vi "Pot Modules.vi"(7 "Console Log in":refnum<class "Console Log.lvclass">, 8 "error in":errorcluster, 11 "Potting Procedure in":refnum<class "Potting Procedure.lvclass">) -> (0 "error out":errorcluster, 3 "Potting Procedure out":refnum<class "Potting Procedure.lvclass">, 5 "Console Log out":refnum<class "Console Log.lvclass">)   [LabVIEW 2011, in "Potting Procedure.lvclass"]
uses:
  Potting Procedure.lvclass
  Application Utilities/Console Log/Console Log.lvclass
  Shared Components/SyringeTool Class/SyringeTool Class.lvclass
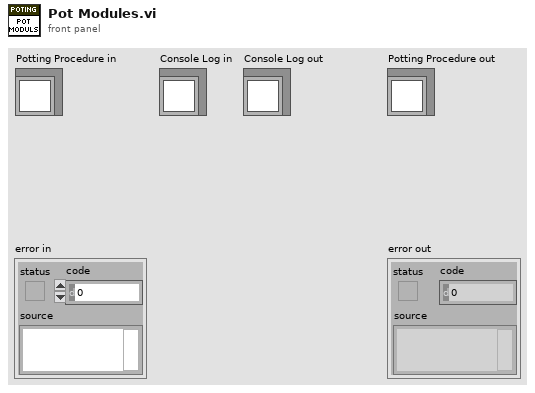
[diagram p1: front panel]
types:
  T1 = typedef "Module Potting Data.ctl" = cluster{"HDI Bond Pad Groups":T2[], "BBM Bond Pad Groups":T2[], "TBM - TBM Side":T2[], "TBM - HDI Side":T2[], "Address Pads":T2[], "Chuck":i32, "Slot":i32, "HV - HDI":T3, "HV - BBM":T3}
  T2 = typedef "3d Line.ctl" = cluster{"Start":refnum<class "Vec3d Class.lvclass">, "End":refnum<class "Vec3d Class.lvclass">, "Enable":bool}
  T3 = typedef "3d Point.ctl" = cluster{"Point":refnum<class "Vec3d Class.lvclass">, "Enable":bool}
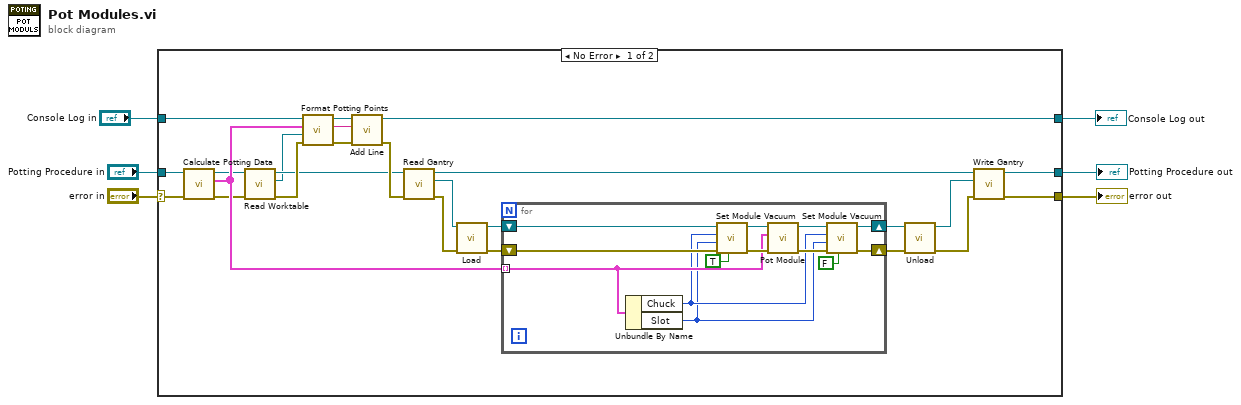
[diagram p0: block diagram]
diagram:
  n1 = case shown="No Error" "error in" {
    selector: "error in" -> [w20 w47]
    tunnel: [w19 w47] -> w5
    tunnel: [w21 w46] -> w3
    tunnel: "Potting Procedure in" -> [w31 w46]
    tunnel: "Console Log in" -> [w18 w45]
    tunnel: [w13 w45] -> w1
    frame No Error {
      n2 = call "Calculate Potting Data.vi"("error in"=w20, "Potting Procedure in"=w31) -> ("error out"=w10:errorcluster, "Module Potting Data"=w17:T1[], "Potting Procedure out"=w11:refnum<class "Potting Procedure.lvclass">)  [unwired: 7 in]
      n3 = call-dynamic "Read Worktable.vi"("error in"=w10, "Potting Procedure in"=w11) -> ("error out"=w9:errorcluster, "WorkTable out"=w7:refnum<class "WorkTable Class.lvclass">, "Potting Procedure out"=w8:refnum<class "Potting Procedure.lvclass">)  [unwired: 7 in]
      n4 = call "Format Potting Points.vi"("error in"=w9, "WorkTable"=w7, "Array"=w17, "Console Log in"=w18) -> ("error out"=w15:errorcluster, "Formatted Potting Points"=w16:string, "Console Log out"=w14:refnum<class "Console Log.lvclass">)  [unwired: 5 in]
      n5 = call "Add Line.vi"("error in"=w15, "String"=w16, "Console Log in"=w14) -> ("error out"=w12:errorcluster, "Console Log out"=w13:refnum<class "Console Log.lvclass">)  [unwired: 7 in]
      n6 = call-dynamic "Read Gantry.vi"("error in (no error)"=w12, "Potting Procedure in"=w8) -> ("error out"=w28:errorcluster, "Gantry"=w30:refnum<class "Gantry Class.lvclass">, "Potting Procedure out"=w25:refnum<class "Potting Procedure.lvclass">)  [unwired: 7 in]
      n7 = call "Load.vi"("error in"=w28, "Gantry in"=w30) -> ("error out"=w27:errorcluster, "SyringeTool out"=w29:refnum<class "SyringeTool Class.lvclass">)  [unwired: 8 in]
      n8 = for {
        tunnel: w17 -> [w35] mode=indexing
        shift-right: [w43] -> w26
        shift-left: w29 -> [w37]
        shift-right: [w41] -> w23
        shift-left: w27 -> [w39]
        n9 = Unbundle By Name(w35) -> ("Chuck"=w34:i32, "Slot"=w33:i32)
        n10 = call-dynamic "Set Module Vacuum.vi"("On/Off"=TRUE, "error in"=w39, "Slot Number"=w33, "Chuck Number"=w34, "Gantry in"=w37) -> ("error out"=w38:errorcluster, "Gantry out"=w36:refnum<class "SyringeTool Class.lvclass">)  [unwired: 5 in]
        n11 = call "Pot Module.vi"("error in"=w38, "Module Potting Data"=w35, "SyringeTool in"=w36) -> ("error out"=w42:errorcluster, "SyringeTool out"=w44:refnum<class "SyringeTool Class.lvclass">)  [unwired: 7 in]
        n12 = call-dynamic "Set Module Vacuum.vi"("On/Off"=FALSE, "error in"=w42, "Slot Number"=w33, "Chuck Number"=w34, "Gantry in"=w44) -> ("error out"=w41:errorcluster, "Gantry out"=w43:refnum<class "SyringeTool Class.lvclass">)  [unwired: 5 in]
      }
      n13 = call "Unload.vi"("error in"=w23, "SyringeTool in"=w26) -> ("error out"=w22:errorcluster, "Gantry out"=w24:refnum<class "Gantry Class.lvclass">)  [unwired: 8 in]
      n14 = call-dynamic "Write Gantry.vi"("error in (no error)"=w22, "Gantry"=w24, "Potting Procedure in"=w25) -> ("error out"=w19:errorcluster, "Potting Procedure out"=w21:refnum<class "Potting Procedure.lvclass">)  [unwired: 7 in]
    }
    frame Error {
    }
  }
  "error out" <- w5
  "Potting Procedure out" <- w3
  "Console Log out" <- w1
